vi "SaveIconToFile.vi"(4 "Image Format":enum32{"PNG", "JPEG", "GIF", "BMP"}(ring), 5 "Image File":path, 6 "error in":errorcluster, 9 "FPWindow in":refnum<class "FPWindow.lvclass">) -> (0 "error out":errorcluster, 3 "FPWindow out":refnum<class "FPWindow.lvclass">)   [LabVIEW 2014, in "Raspberry Pi Compatible Compiler for LabVIEW.lvlib" / "FPWindow.lvclass"]
uses:
  FPWindow.lvclass
  FPWindow.lvclass/FPWindow.ctl
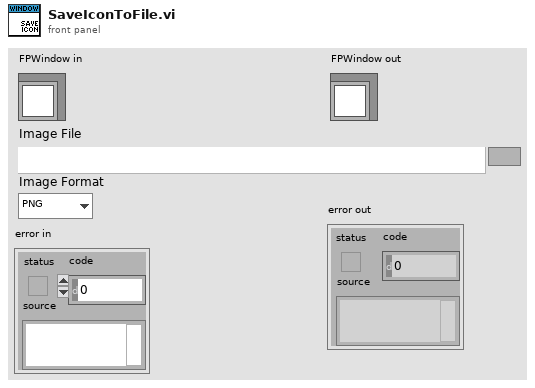
[diagram p1: front panel]
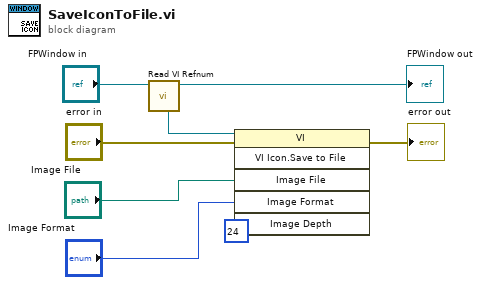
[diagram p0: block diagram]
diagram:
  n1 = call "Read VI Refnum.vi"("FPWindow in"="FPWindow in") -> ("FPWindow out"=→"FPWindow out":refnum<class "FPWindow.lvclass">, "VI Refnum"=w7:refnum<vi>)  [unwired: 7 in]
  n2 = invoke class="VI" method="VI Icon.Save to File"(reference=w7, error in="error in", "Image File"="Image File", "Image Format"="Image Format", "Image Depth"=24) -> (error out=→"error out":errorcluster)  [unwired: 1 in, 5 out]
